vi "Subvi gated pixel clock generator.vi"(9 "Nmax lines":u16) -> ()   [LabVIEW 2017]
uses:
  <vilib>/Platform/TimedLoop/XDataNode/timing_clust.ctl
  <vilib>/Platform/TimedLoop/XDataNode/nitl_modes.ctl
  <vilib>/Platform/TimedLoop/XDataNode/wakeup.ctl
  <vilib>/rvi/Emulation/niFpgaSctlEmulationGetInTimedLoop.vi
  <vilib>/rvi/Emulation/niFpgaEmulationReportErrorSimple.vi
  <vilib>/rvi/Emulation/niFpgaGetClockAttributes.vi
  <vilib>/rvi/Emulation/niFpgaCriticalErrorInLSC.vi
  <vilib>/rvi/Emulation/niFpgaProcessEmulError.vi
  GV pixel clock.vi
  GV line clock change.vi
  <vilib>/Platform/TimedLoop/XDataNode/XDataNode.xnode
  <vilib>/Platform/TimedLoop/XDataNode/XDNodeRunTimeDep.lvlib
  GV gated pixel clock change.vi
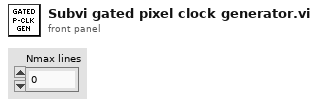
[diagram p1: front panel]
types:
  T1 = typedef "XDNodeRunTimeDep.lvlib/timing_clust.ctl" = cluster{"Expected End [f-1]":u64, "Actual End [f-1]":u64, "Finished Late? [f-1]":bool, "Expected End [i-1]":u64, "Actual End [i-1]":u64, "Finished Late? [i-1]":bool, "Expected Start [i]":u64, "Actual Start [i]":u64, "Expected Start [f]":u64, "Actual Start [f]":u64, "Source Name":string, "Structure Name":string, "Period":i64, "Deadline":i64, "Offset":i64, "Start":i64, "Priority":i32, "Timeout":i32, "Mode":T2, "Wakeup Reason":T3, "Error":errorcluster, "Source Type":string, "Secondary Source Type":string, "Global End Time":u64, "Global Start Time":u64, "Frame Duration":u64, "Iteration Duration":u64, "Assigned CPU":i32, "I/O Scan Engine Mode":u32}
  T2 = typedef "XDNodeRunTimeDep.lvlib/nitl_modes.ctl" = enum32{"No Change", "Process missed periods, maintain original phase", "Discard missed periods, maintain original phase", "Process missed periods, ignore original phase", "Discard missed periods, ignore original phase"}
  T3 = typedef "XDNodeRunTimeDep.lvlib/wakeup.ctl" = enum32{"Normal", "Aborted", "Asynchronous wakeup", "Timing source error", "Timed loop error", "Timeout"}
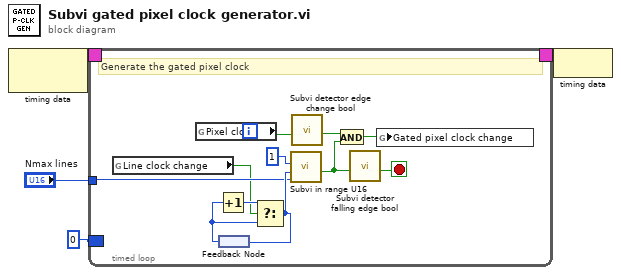
[diagram p0: block diagram]
diagram:
  n1 = node-c288() -> (w4:T1)  [unwired: 1 in]
  n2 = timed-loop {
    timing: w4 -> [_]
    timing-out: [_] -> w3
    tunnel: "Nmax lines" -> [w10]
    border: u16 0 -> [_]
    stop <- w7 stop-if-true
    # "Generate the gated pixel clock"
    n3 = global read "GV line clock change.vi" "Line clock change"() -> (w9:bool)
    n4 = global read "GV pixel clock.vi" "Pixel clock"() -> (w5:bool)
    n5 = feedback #1() -> (w6:u16)
    n6 = Increment(x=w6) -> (x+1=w11:u16)
    n7 = Select(t=w11, s=w9, f=w6) -> (s? t:f=w12:u16)
    n8 = feedback-in #1(w12) -> ()
    n9 = call "Subvi in range U16.vi"("Max"=w10, "Input"=w12, "Min"=u16 1) -> ("In range"=w8:bool)  [unwired: 8 in]
    n10 = call "Subvi detector edge change bool.vi"("Input"=w5) -> ("Output"=w15:bool)  [unwired: 8 in]
    n11 = And(x=w15, y=w8) -> (x .and. y?=w14:bool)
    n12 = call "Subvi detector falling edge bool.vi"("Input"=w8) -> ("Output"=w7:bool)  [unwired: 10 in]
    n13 = global write "GV gated pixel clock change.vi" "Gated pixel clock change"(w14) -> ()
  }
  n14 = node-c288(w3) -> ()
